vi "moving_button.vi"() -> ()   [LabVIEW 2021]
panel:
  in  "stop":bool
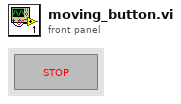
[diagram p1: front panel]
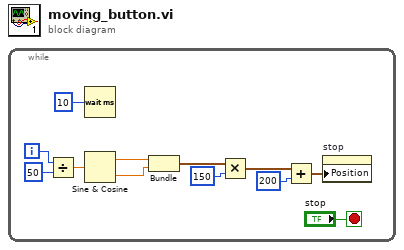
[diagram p0: block diagram]
diagram:
  n1 = while {
    i -> [w11]
    stop <- "stop" stop-if-true
    n2 = Divide(x=w11, y=50) -> (x/y=w10:dbl)
    n3 = Wait (ms)(milliseconds to wait=u32 10) -> ()  [unwired: 1 out]
    n4 = Sine & Cosine(0:w10) -> (1:w7:dbl, 2:w6:dbl)
    n5 = Bundle(w7, w6) -> (w5:cluster{dbl, dbl})  [unwired: 1 in]
    n6 = Multiply(x=w5, y=150) -> (x*y=w3:cluster{dbl, dbl})
    n7 = Add(x=w3, y=200) -> (x+y=w1:cluster{dbl, dbl})
    n8 = property on="stop" class="Bool"("Position"=w1) -> ()  [unwired: 2 in, 2 out]
  }
